vi "Stop Core.vi"(10 "final error code":i32, 11 "UI in":refnum<class "UI.lvclass">) -> (3 "UI out":refnum<class "UI.lvclass">)   [LabVIEW 2016, in "Generic UI Actor.lvlib" / "UI.lvclass"]
uses:
  <userlib>/Common Components/User Interface/UI.lvclass
  C:/Program Files (x86)/National Instruments/LabVIEW 2016/vi.lib/ActorFramework/Actor/Actor.lvclass
  <vilib>/ActorFramework/Actor/Actor.lvclass/Actor.ctl
  <userlib>/Common Components/User Interface/UI.lvclass/UI.ctl
  <vilib>/ActorFramework/Message Enqueuer/Message Enqueuer.lvclass/Message Enqueuer.ctl
  <userlib>/Common Components/User Interface/Accessors/Read This VI.vi
  <vilib>/ActorFramework/Message Enqueuer/Enqueue.vi
  <vilib>/ActorFramework/Stop Msg/Stop Msg.lvclass
  C:/Program Files (x86)/National Instruments/LabVIEW 2016/vi.lib/ActorFramework/Message/Message.lvclass
  <vilib>/ActorFramework/Message Priority Queue/Priority Enqueue.vi
  <vilib>/ActorFramework/Actor/Actor.lvclass
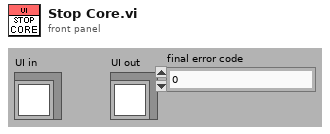
[diagram p1: front panel]
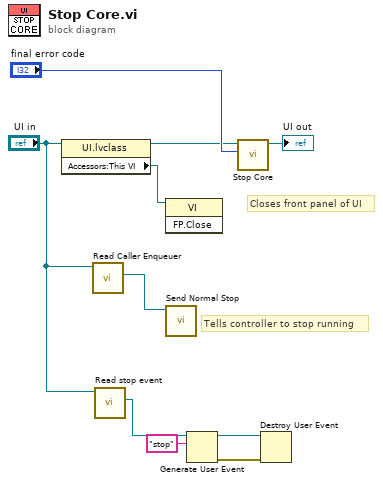
[diagram p0: block diagram]
diagram:
  # "Closes front panel of UI"
  # "Tells controller to stop running"
  n1 = property class="UI.lvclass"(reference="UI in") -> (reference out=w2:refnum<class "UI.lvclass">, "Accessors:This VI"=w1:refnum<vi>)  [unwired: 1 in, 1 out]
  n2 = call <vilib>:"Read Caller Enqueuer.vi"("Actor"="UI in") -> ("Caller Enqueuer"=w9:refnum<class "Message Enqueuer.lvclass">)  [unwired: 10 in]
  n3 = call <userlib>:"Read stop event.vi"("UI in"="UI in") -> ("stop event"=w5:refnum<user-event>)  [unwired: 8 in, 2 out]
  n4 = invoke class="VI" method="FP.Close"(reference=w1) -> ()  [unwired: 2 in, 3 out]
  n5 = call <vilib>:"Send Normal Stop.vi"("Message Enqueuer"=w9) -> ()  [unwired: 10 in, 1 out]
  n6 = Generate User Event(user event=w5, event data cluster="stop" ("event data")) -> (user event out=w7:refnum<user-event>, error out=w6:errorcluster)  [unwired: 2 in]
  n7 = call-parent "Stop Core.vi"("final error code"="final error code", "Actor in"=w2) -> ("Actor out"=→"UI out":refnum<class "UI.lvclass">)  [unwired: 9 in]
  n8 = Destroy User Event(user event=w7, error in=w6) -> ()  [unwired: 1 out]
